vi "favicon.ico.vi"(9 "Body Data":string, 10 "Form Data":cluster{"key":string[], "value":string[]}, 11 "Method":string) -> (3 "Content":string)   [LabVIEW 2019, in "HTTP Server.lvlib"]
uses:
  HTTP Server.lvlib
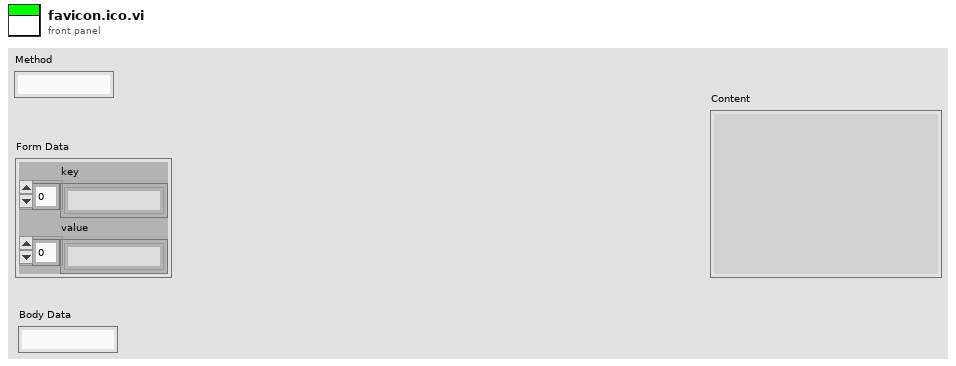
[diagram p1: front panel]
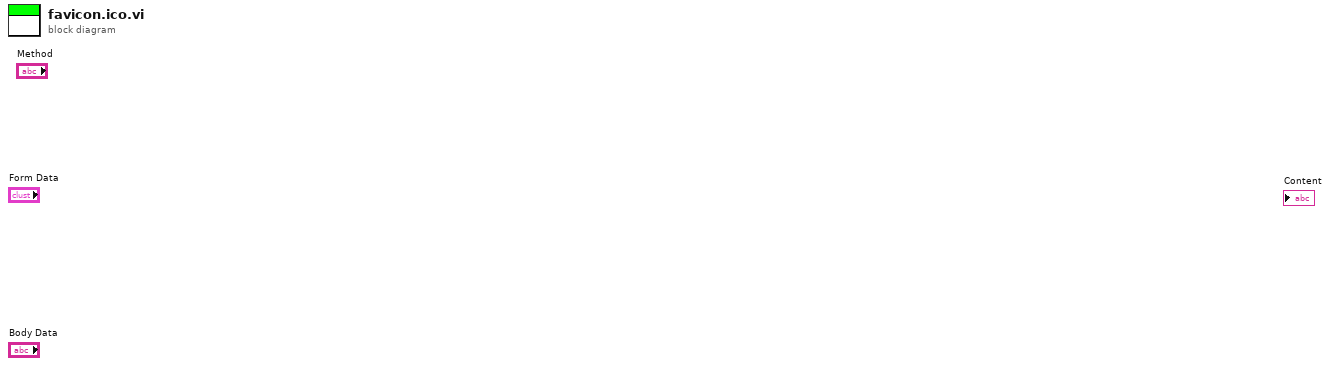
[diagram p0: block diagram]
diagram:
